vi "IPX_HTTP_test.vi"() -> ()   [LabVIEW 2014, in "IPX_HTTP.lvlib"]
uses:
  IPX_HTTP.lvlib
panel:
  in  "Value":enum16{"0", "1"}(ring)
  in  "Value to write":bool
  in  "Write":bool
  out "Waveform Chart":i16(graph)
  in  "Stop Button":bool
  in  "Play Button":bool
  out "Error Out":errorcluster
  in  "Error In":errorcluster
  out "Value":i16
  in  "Way":u16(ring) items=["1", "2", "3", "4", "5", "6", "7", "8"]
  in  "Port (80-8000)":dbl=80.0
  in  "IP adress (XXX.XXX.XXX.XXX)":string
  in  "Mesure type":T1(ring)
  # "IPX-800 Test"
  # "CONNECTION"
  # "RESULTS"
  # "SETTINGS"
  # "Please visit http://www.OpenG.org to learn about the\nOpen Source LabVIEW software movement.\n\nNOTICE -- YOU MUST LEAVE THIS NOTICE IN PLACE.  PER THE TERMS OF THE LICENSE BELOW, YOU MAY SUBLICENSE THIS SOFTWARE\nIN ANY WAY THAT DOES NOT CONFLICT WITH THIS LICENSE.\n\n### BSD License (http://www.opensource.org/licenses/bsd-license.php) Begin ###\n\nCopyright (c) 2014, Emmanuel Landrivon <emmanuel.landrivon@ircelyon.univ-lyon1.fr>\nFlorian Chapon <florian.chapon@ircelyon.univ-lyon1.fr\n\n\nAll rights reserved.\n\nRedistribution and use in source and binary forms, with or without modification, are permitted provided that the following conditions are met:\n\n    * Redistributions of source code must retain the above copyright notice, this list of conditions and the following disclaimer.\n    * Redistributions in binary form must reproduce the above copyright notice, this list of conditions and the following disclaimer in the\n       documentation and/or other materials provided with the distribution.\n  \nTHIS SOFTWARE IS PROVIDED BY THE COPYRIGHT HOLDERS AND CONTRIBUTORS \"AS IS\" AND ANY EXPRESS OR IMPLIED WARRANTIES,\nINCLUDING, BUT NOT LIMITED TO, THE IMPLIED WARRANTIES OF MERCHANTABILITY AND FITNESS FOR A PARTICULAR PURPOSE ARE\nDISCLAIMED. IN NO EVENT SHALL THE COPYRIGHT OWNER OR CONTRIBUTORS BE LIABLE FOR ANY DIRECT, INDIRECT, INCIDENTAL,\nSPECIAL, EXEMPLARY, OR CONSEQUENTIAL DAMAGES (INCLUDING, BUT NOT LIMITED TO, PROCUREMENT OF SUBSTITUTE GOODS OR\nSERVICES; LOSS OF USE, DATA, OR PROFITS; OR BUSINESS INTERRUPTION) HOWEVER CAUSED AND ON ANY THEORY OF LIABILITY,\nWHETHER IN CONTRACT, STRICT LIABILITY, OR TORT (INCLUDING NEGLIGENCE OR OTHERWISE) ARISING IN ANY WAY OUT OF THE USE\nOF THIS SOFTWARE, EVEN IF ADVISED OF THE POSSIBILITY OF SUCH DAMAGE.\n\n### BSD License End ###"
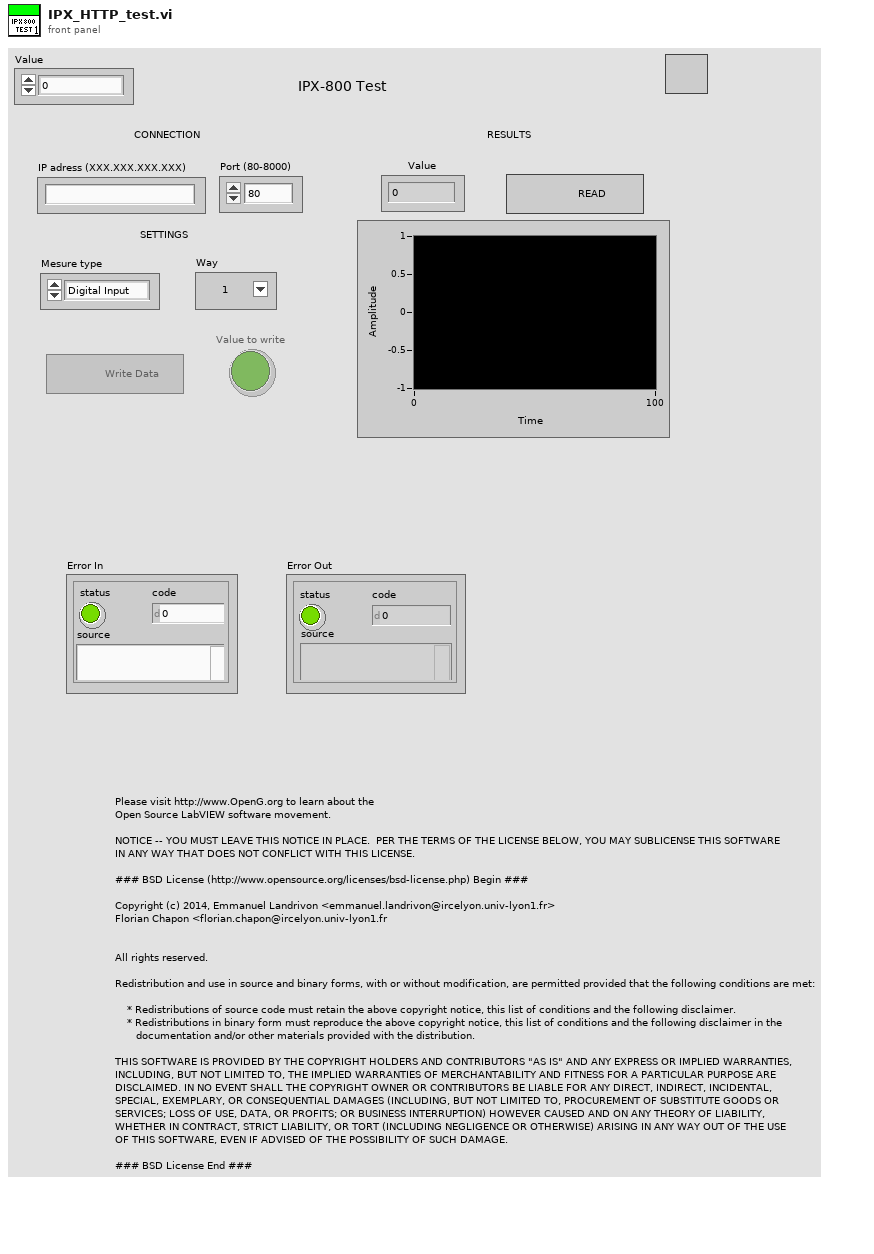
[diagram p1: front panel]
types:
  T1 = enum16{"Digital Input", "Digital Output", "Analog Input"}
  T2 = enum8{"Enabled", "Disabled", "Disabled and Grayed Out"}
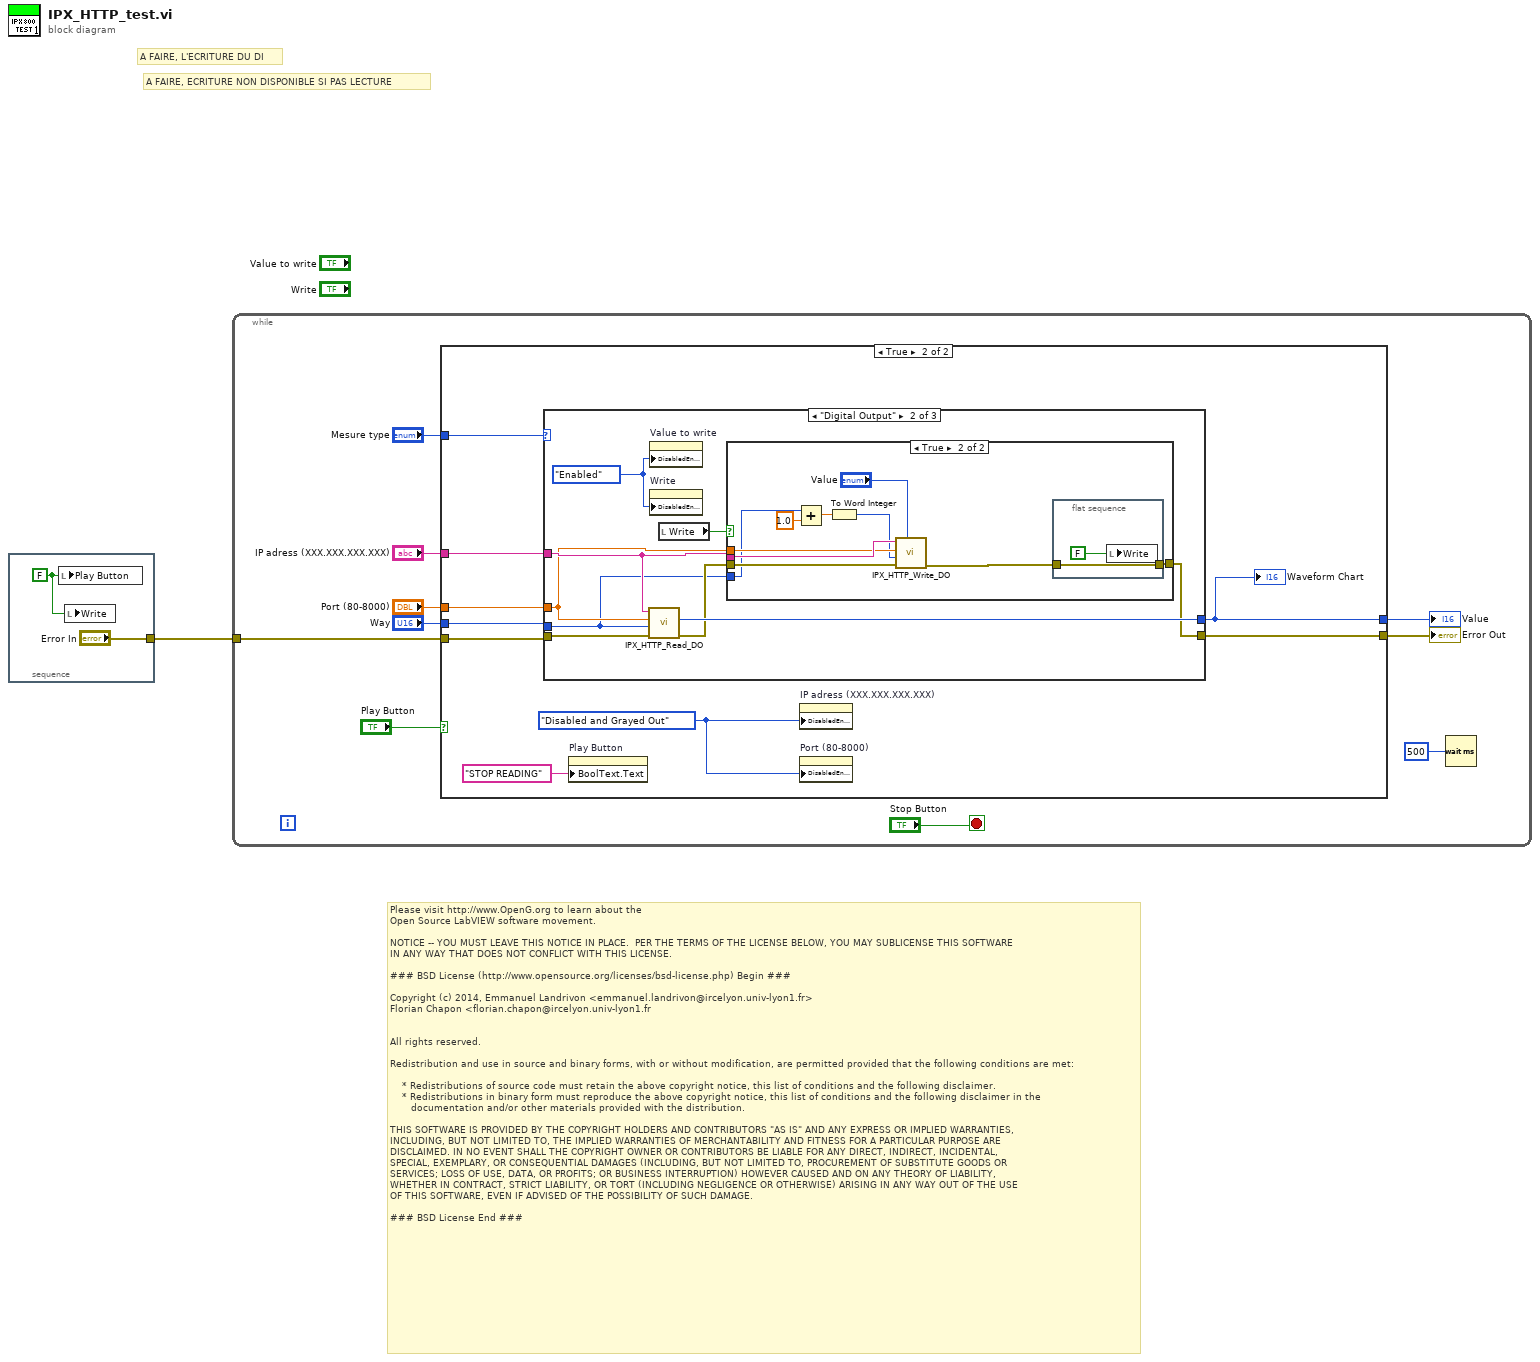
[diagram p0: block diagram]
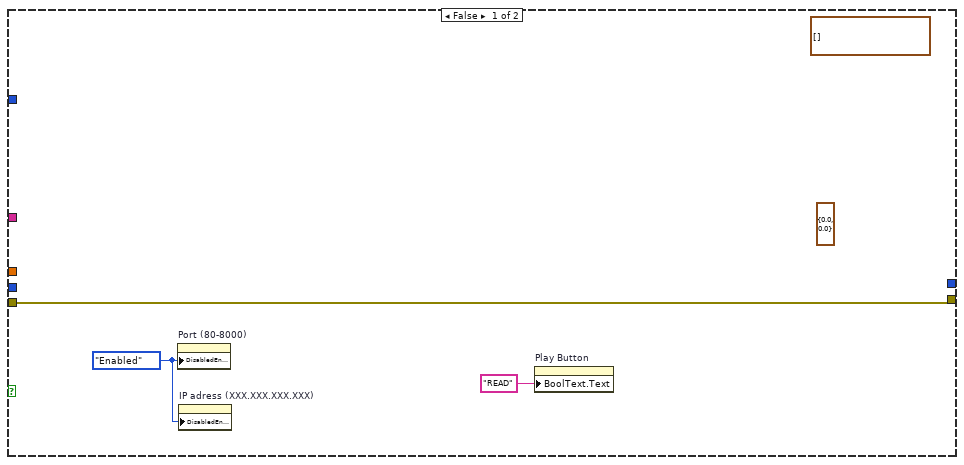
[diagram p2: hidden frame]
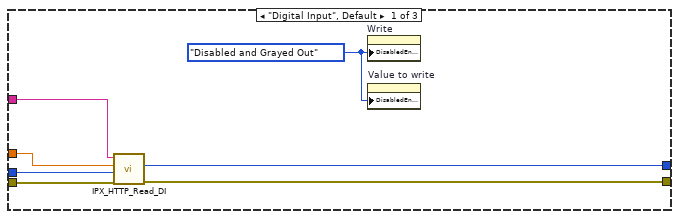
[diagram p3: hidden frame]
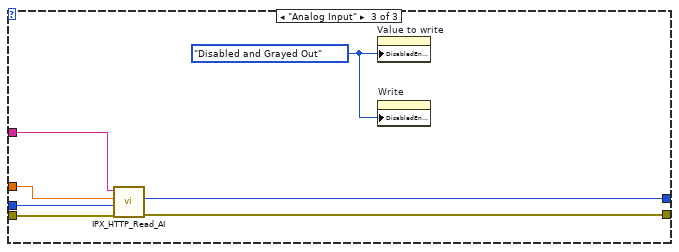
[diagram p5: hidden frame]
diagram:
  # "Please visit http://www.OpenG.org to learn about the\nOpen Source LabVIEW software movement.\n\nNOTICE -- YOU MUST LEAVE THIS NOTICE IN PLACE.  PER THE TERMS OF THE LICENSE BELOW, YOU MAY SUBLICENSE THIS SOFTWARE\nIN ANY WAY THAT DOES NOT CONFLICT WITH THIS LICENSE.\n\n### BSD License (http://www.opensource.org/licenses/bsd-license.php) Begin ###\n\nCopyright (c) 2014, Emmanuel Landrivon <emmanuel.landrivon@ircelyon.univ-lyon1.fr>\nFlorian Chapon <florian.chapon@ircelyon.univ-lyon1.fr\n\n\nAll rights reserved.\n\nRedistribution and use in source and binary forms, with or without modification, are permitted provided that the following conditions are met:\n\n    * Redistributions of source code must retain the above copyright notice, this list of conditions and the following disclaimer.\n    * Redistributions in binary form must reproduce the above copyright notice, this list of conditions and the following disclaimer in the\n       documentation and/or other materials provided with the distribution.\n  \nTHIS SOFTWARE IS PROVIDED BY THE COPYRIGHT HOLDERS AND CONTRIBUTORS \"AS IS\" AND ANY EXPRESS OR IMPLIED WARRANTIES,\nINCLUDING, BUT NOT LIMITED TO, THE IMPLIED WARRANTIES OF MERCHANTABILITY AND FITNESS FOR A PARTICULAR PURPOSE ARE\nDISCLAIMED. IN NO EVENT SHALL THE COPYRIGHT OWNER OR CONTRIBUTORS BE LIABLE FOR ANY DIRECT, INDIRECT, INCIDENTAL,\nSPECIAL, EXEMPLARY, OR CONSEQUENTIAL DAMAGES (INCLUDING, BUT NOT LIMITED TO, PROCUREMENT OF SUBSTITUTE GOODS OR\nSERVICES; LOSS OF USE, DATA, OR PROFITS; OR BUSINESS INTERRUPTION) HOWEVER CAUSED AND ON ANY THEORY OF LIABILITY,\nWHETHER IN CONTRACT, STRICT LIABILITY, OR TORT (INCLUDING NEGLIGENCE OR OTHERWISE) ARISING IN ANY WAY OUT OF THE USE\nOF THIS SOFTWARE, EVEN IF ADVISED OF THE POSSIBILITY OF SUCH DAMAGE.\n\n### BSD License End ###"
  # "A FAIRE, ECRITURE NON DISPONIBLE SI PAS LECTURE"
  # "A FAIRE, L'ECRITURE DU DI"
  n1 = stacked-sequence {
    tunnel: ["Error In"] -> w1
    frame #0 {
      w3 = FALSE ("Play Button")
      n2 = local write "Play Button"(w3) -> ()
      n3 = local write "Write"(w3) -> ()
    }
  }
  n4 = while {
    tunnel: w1 -> [w4]
    stop <- "Stop Button" stop-if-true
    n5 = case shown="True" "Play Button" {
      tunnel: "Mesure type" -> [_ w18]
      tunnel: "IP adress (XXX.XXX.XXX.XXX)" -> [_ w19]
      tunnel: "Port (80-8000)" -> [_ w25]
      tunnel: [_ w20] -> w5
      tunnel: [w16 w17] -> w11
      tunnel: w4 -> [w16 w24]
      tunnel: "Way" -> [_ w23]
      frame False {
        (unwired) timestamp[] []
        (unwired) cluster{dbl, dbl} {0.0, 0.0}
        w15 = T2."Enabled" ("Disabled")
        n6 = property on="Port (80-8000)" class="DigNum (strict)"("DisabledEnum"=w15) -> ()  [unwired: 2 in, 2 out]
        n7 = property on="IP adress (XXX.XXX.XXX.XXX)" class="Str"("DisabledEnum"=w15) -> ()  [unwired: 2 in, 2 out]
        n8 = property on="Play Button" class="Bool (strict)"("BoolText.Text"="READ" ("Boolean Text.Text")) -> ()  [unwired: 2 in, 2 out]
      }
      frame True {
        w22 = T2."Disabled and Grayed Out" ("Disabled")
        n9 = case shown="\"Digital Output\"" w18 {
          tunnel: w19 -> [w30 w38 w61]
          tunnel: w25 -> [w29 w37 w60]
          tunnel: w23 -> [w28 w36 w59]
          tunnel: [w31 w40 w58] -> w20
          tunnel: [w27 w35 w57] -> w17
          tunnel: w24 -> [w32 w41 w56]
          frame "Digital Input", Default {
            w26 = T2."Disabled and Grayed Out" ("Disabled")
            n10 = call "IPX_HTTP_Read_DI.vi"("Error In"=w32, "Voie"=w28, "Port (80-8000)"=w29, "IP adress (XXX.XXX.XXX.XXX)"=w30) -> ("Error Out"=w27:errorcluster, "Value"=w31:i16)  [unwired: 6 in]
            n11 = property on="Write" class="Bool (strict)"("DisabledEnum"=w26) -> ()  [unwired: 2 in, 2 out]
            n12 = property on="Value to write" class="Bool (strict)"("DisabledEnum"=w26) -> ()  [unwired: 2 in, 2 out]
          }
          frame "Digital Output" {
            w33 = T2."Enabled" ("Disabled")
            n13 = call "IPX_HTTP_Read_DO.vi"("Error In"=w41, "Voie"=w36, "Port (80-8000)"=w37, "IP adress (XXX.XXX.XXX.XXX)"=w38) -> ("Error Out"=w39:errorcluster, "Value"=w40:i16)  [unwired: 6 in]
            n14 = property on="Value to write" class="Bool (strict)"("DisabledEnum"=w33) -> ()  [unwired: 2 in, 2 out]
            n15 = property on="Write" class="Bool (strict)"("DisabledEnum"=w33) -> ()  [unwired: 2 in, 2 out]
            n16 = local read "Write"() -> (w34:bool)
            n17 = case shown="True" w34 {
              tunnel: w38 -> [_ w52]
              tunnel: w37 -> [_ w51]
              tunnel: w39 -> [w42 w50]
              tunnel: [w42 w44] -> w35
              tunnel: w36 -> [_ w48]
              frame False {
              }
              frame True {
                n18 = Add(x=w48, y=1.0) -> (x+y=w47:dbl)
                n19 = To Word Integer(number=w47) -> (16bit integer=w46:i16)
                n20 = call "IPX_HTTP_Write_DO.vi"("Value"="Value", "Error In"=w50, "Digital Output"=w46, "Port (80-8000)"=w51, "IP adress (XXX.XXX.XXX.XXX)"=w52) -> ("Error Out"=w45:errorcluster)  [unwired: 6 in]
                n21 = flat-sequence {
                  tunnel: w45 -> [w53]
                  tunnel: [w53] -> w44
                  frame #0 {
                    n22 = local write "Write"(FALSE ("Write")) -> ()
                  }
                }
              }
            }
          }
          frame "Analog Input" {
            w55 = T2."Disabled and Grayed Out" ("Disabled")
            n23 = call "IPX_HTTP_Read_AI.vi"("Error In"=w56, "Voie"=w59, "Port (80-8000)"=w60, "IP adress (XXX.XXX.XXX.XXX)"=w61) -> ("Error Out"=w57:errorcluster, "Value"=w58:i16)  [unwired: 6 in]
            n24 = property on="Value to write" class="Bool (strict)"("DisabledEnum"=w55) -> ()  [unwired: 2 in, 2 out]
            n25 = property on="Write" class="Bool (strict)"("DisabledEnum"=w55) -> ()  [unwired: 2 in, 2 out]
          }
        }
        "Waveform Chart" <- w20
        n26 = property on="Play Button" class="Bool (strict)"("BoolText.Text"="STOP READING" ("Boolean Text.Text")) -> ()  [unwired: 2 in, 2 out]
        n27 = property on="IP adress (XXX.XXX.XXX.XXX)" class="Str"("DisabledEnum"=w22) -> ()  [unwired: 2 in, 2 out]
        n28 = property on="Port (80-8000)" class="DigNum (strict)"("DisabledEnum"=w22) -> ()  [unwired: 2 in, 2 out]
      }
    }
    "Value" <- w5
    "Error Out" <- w11
    n29 = Wait (ms)(milliseconds to wait=u32 500) -> ()  [unwired: 1 out]
  }
